vi "Destroy.vi"(8 "error in (no error)":errorcluster, 11 "reference in":refnum<class "WebSocket.lvclass">) -> (0 "error out":errorcluster, 3 "reference out":refnum<class "WebSocket.lvclass">)   [LabVIEW 2017, in "WebSocket.lvclass"]
uses:
  WebSocket.lvclass
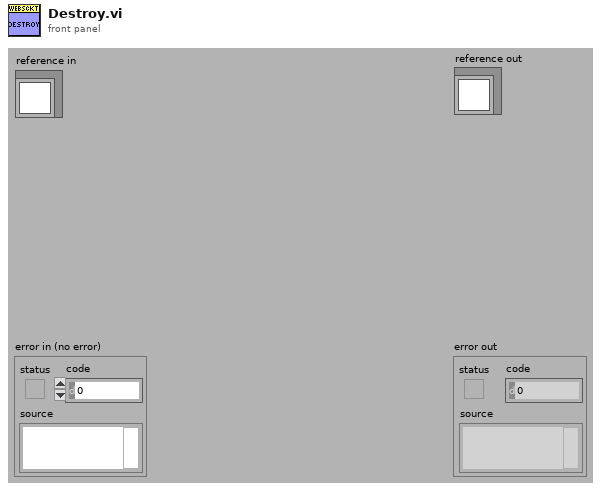
[diagram p1: front panel]
types:
  T1 = typedef "WebSocket.lvclass/ObjectAttributes.ctl" = cluster{"Socket":refnum<k5>, "Thread":refnum<vi>, "From Socket":refnum<queue>, "To Socket":refnum<queue>, "Rx Stats in Progress":variant, "Rx Stats":variant, "Tx Stats in Progress":variant, "Tx Stats":variant}
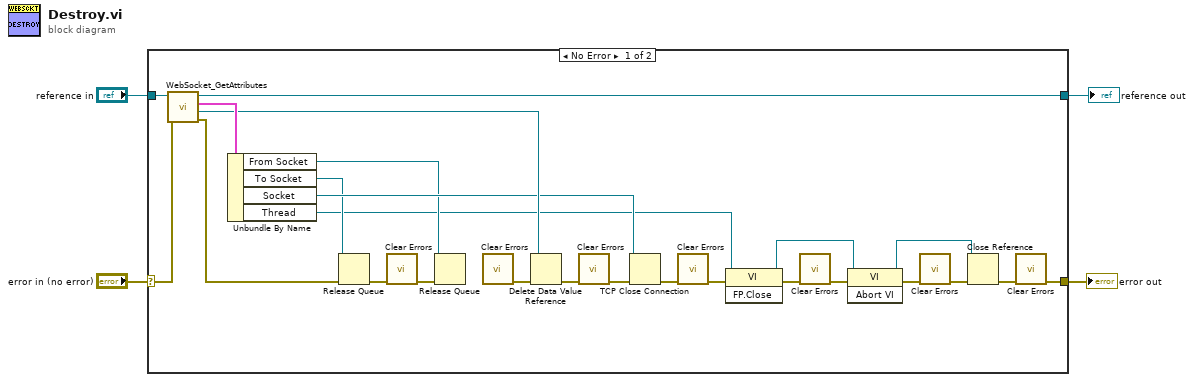
[diagram p0: block diagram]
diagram:
  n1 = case shown="No Error" "error in (no error)" {
    selector: "error in (no error)" -> [w28 w31]
    tunnel: [w5 w31] -> w1
    tunnel: [w25 w30] -> w2
    tunnel: "reference in" -> [w29 w30]
    frame No Error {
      n2 = call "WebSocket_GetAttributes.vi"("error in (no error)"=w28, "reference in"=w29) -> ("error out"=w8:errorcluster, "DataRef"=w26:refnum<data-value>, "Data"=w27:T1, "reference out"=w25:refnum<class "WebSocket.lvclass">)  [unwired: 6 in]
      n3 = Unbundle By Name(w27) -> ("From Socket"=w10:refnum<queue>, "To Socket"=w11:refnum<queue>, "Socket"=w15:refnum<k5>, "Thread"=w9:refnum<vi>)
      n4 = Release Queue(queue=w11, error in (no error)=w8) -> (error out=w12:errorcluster)  [unwired: 1 in, 2 out]
      n5 = call <vilib>:"Clear Errors.vi"("error in (no error)"=w12) -> ("error out"=w13:errorcluster)  [unwired: 5 in, 1 out]
      n6 = Release Queue(queue=w10, error in (no error)=w13) -> ()  [unwired: 1 in, 3 out]
      n7 = call <vilib>:"Clear Errors.vi"() -> ("error out"=w14:errorcluster)  [unwired: 6 in, 1 out]
      n8 = Delete Data Value Reference(data value reference=w26, error in=w14) -> (error out=w24:errorcluster)  [unwired: 1 out]
      n9 = call <vilib>:"Clear Errors.vi"("error in (no error)"=w24) -> ("error out"=w7:errorcluster)  [unwired: 5 in, 1 out]
      n10 = TCP Close Connection(connection ID=w15, error in (no error)=w7) -> (error out=w16:errorcluster)  [unwired: 1 in, 1 out]
      n11 = call <vilib>:"Clear Errors.vi"("error in (no error)"=w16) -> ("error out"=w6:errorcluster)  [unwired: 5 in, 1 out]
      n12 = invoke class="VI" method="FP.Close"(reference=w9, error in=w6) -> (reference out=w20:refnum<vi>, error out=w21:errorcluster)  [unwired: 1 in, 1 out]
      n13 = call <vilib>:"Clear Errors.vi"("error in (no error)"=w21) -> ("error out"=w17:errorcluster)  [unwired: 5 in, 1 out]
      n14 = invoke class="VI" method="Abort VI"(reference=w20, error in=w17) -> (reference out=w19:refnum<vi>, error out=w22:errorcluster)  [unwired: 1 in, 1 out]
      n15 = call <vilib>:"Clear Errors.vi"("error in (no error)"=w22) -> ("error out"=w18:errorcluster)  [unwired: 5 in, 1 out]
      n16 = Close Reference(reference=w19, error in (no error)=w18) -> (error out=w23:errorcluster)
      n17 = call <vilib>:"Clear Errors.vi"("error in (no error)"=w23) -> ("error out"=w5:errorcluster)  [unwired: 5 in, 1 out]
    }
    frame Error {
    }
  }
  "error out" <- w1
  "reference out" <- w2
